vi "dfd_Polynomial Trail Zero Remover.vi"(1 "tol":dbl=1e-12 min=0.0 step=1e-12 format="%.2e", 2 "poly in":dbl[](array[numeric]) format="%.2f") -> (0 "poly out":dbl[](array[numeric]) format="%.2f")   [LabVIEW 2017, in "NI_DigFilterLicensed.lvlib"]
uses:
  <vilib>/addons/Digital Filter Design/NI_DigFilterLicensed.lvlib
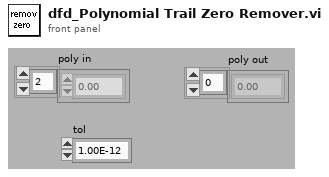
[diagram p1: front panel]
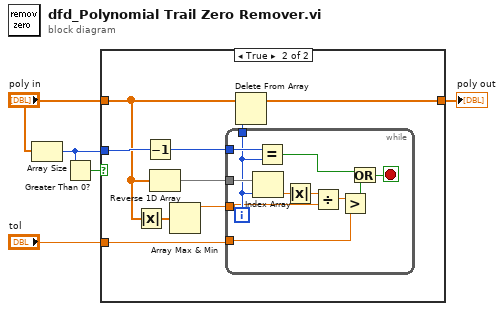
[diagram p0: block diagram]
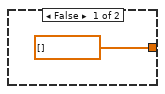
[diagram p2: hidden frame]
diagram:
  n1 = Array Size(array="poly in") -> (size(s)=w2:i32)
  n2 = Greater Than 0?(x=w2) -> (x > 0?=w3:bool)
  n3 = case shown="True" w3 {
    tunnel: "poly in" -> [_ w9]
    tunnel: [dbl[] [] w13] -> w4
    tunnel: w2 -> [_ w11]
    tunnel: "tol" -> [_ w12]
    frame False {
    }
    frame True {
      n4 = Absolute Value(x=w9) -> (abs(x)=w8:dbl[])
      n5 = Decrement(x=w11) -> (x-1=w10:i32)
      n6 = Reverse 1D Array(array=w9) -> (reversed array=w15:dbl[])
      n7 = Array Max & Min(array=w8) -> (max value=w7:dbl)  [unwired: 3 out]
      n8 = while {
        tunnel: w15 -> [w26]
        tunnel: w10 -> [w25]
        tunnel: [w22] -> w14
        tunnel: w12 -> [w19]
        tunnel: w7 -> [w17]
        i -> [w22]
        stop <- w23 stop-if-true
        n9 = Index Array(array=w26, index=w22) -> (element=w21:dbl)
        n10 = Equal?(x=w25, y=w22) -> (x = y?=w24:bool)
        n11 = Absolute Value(x=w21) -> (abs(x)=w18:dbl)
        n12 = Divide(x=w18, y=w17) -> (x/y=w16:dbl)
        n13 = Greater?(x=w16, y=w19) -> (0:w20:bool)
        n14 = Or(x=w24, y=w20) -> (x .or. y?=w23:bool)
      }
      n15 = Delete From Array(array=w9, length=w14) -> (array with subset deleted=w13:dbl[])  [unwired: 1 in, 1 out]
    }
  }
  "poly out" <- w4
